vi "Dynamic Position Maths.vi"(0 "Height(%)":dbl, 5 "Width(%)":dbl, 9 "Position":T1, 11 "error in (no error)":errorcluster, 12 "Left Offset (%)":dbl, 13 "Top Offset (%)":dbl) -> (4 "Height":u32, 6 "Width":u32, 8 "Position Out":T1, 10 "Start Pos of next control":T1, 15 "error out":errorcluster)   [LabVIEW 2014]
uses:
  <vilib>/Utility/miscctls.llb/LVPositionTypeDef.ctl
panel:
  out "Bottom":u32
  out "Right":u32
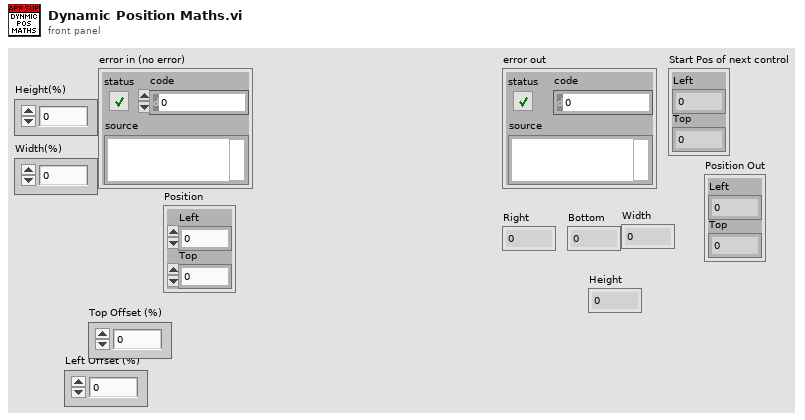
[diagram p1: front panel]
types:
  T1 = typedef "LVPositionTypeDef.ctl" = cluster{"Left":i32, "Top":i32}
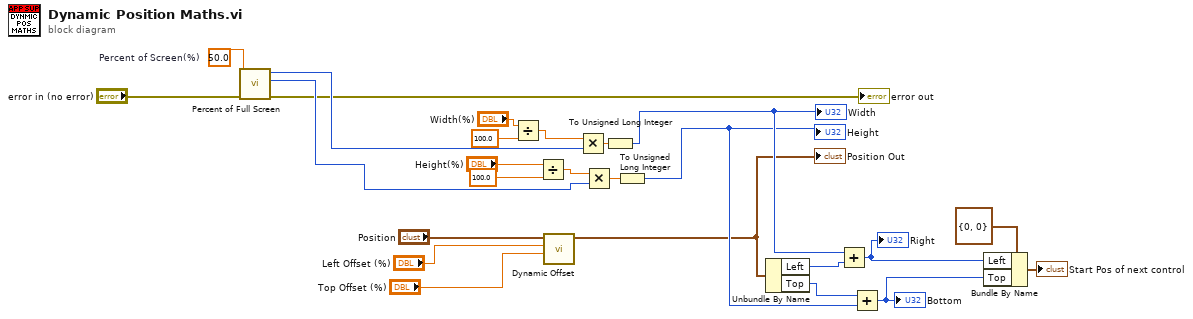
[diagram p0: block diagram]
diagram:
  w1 = 50.0  # Percent of Screen(%)
  n1 = call "Percent of Full Screen.vi"("error in (no error)"="error in (no error)", 11:w1) -> ("error out"=→"error out":errorcluster, "Bottom"=w4:i16, "Right"=w5:i16)  [unwired: 7 in]
  n2 = Divide(x="Width(%)", y=100.0) -> (x/y=w23:dbl)
  n3 = Divide(x="Height(%)", y=100.0) -> (x/y=w20:dbl)
  n4 = call "Dynamic Offset.vi"("Top Offset (%)"="Top Offset (%)", "Left Offset (%)"="Left Offset (%)", "Position"="Position") -> ("Offset Positon"=w6:T1)  [unwired: 7 in, 1 out]
  "Position Out" <- w6
  n5 = Multiply(x=w23, y=w5) -> (x*y=w19:dbl)
  n6 = Multiply(x=w20, y=w4) -> (x*y=w18:dbl)
  n7 = To Unsigned Long Integer(number=w19) -> (unsigned 32bit integer=w16:u32)
  "Width" <- w16
  n8 = To Unsigned Long Integer(number=w18) -> (unsigned 32bit integer=w14:u32)
  "Height" <- w14
  n9 = Unbundle By Name(w6) -> ("Left"=w17:i32, "Top"=w15:i32)
  n10 = Add(x=w16, y=w17) -> (x+y=w12:u32)
  "Right" <- w12
  n11 = Add(x=w15, y=w14) -> (x+y=w11:u32)
  "Bottom" <- w11
  n12 = Bundle By Name(cluster=T1 {"Left"=0, "Top"=0} ("Position"), "Left"=w12, "Top"=w11) -> (→"Start Pos of next control":T1)
